vi "Read Std Dev.vi"(8 "error in (no error)":errorcluster, 11 "Std Dev in":refnum<class "Std Dev.lvclass">) -> (0 "error out":errorcluster, 1 "Channels w/ Std Dev":string[](array[string]), 2 "4 Data Points":dbl[](array[numeric]), 3 "Std Dev out":refnum<class "Std Dev.lvclass">)   [LabVIEW 2009, in "Std Dev.lvclass"]
doc: "Returns the Standard Deviation of a readable instrument.\n\nPublic Interface for \"_Read.vi\""
uses:
  Std Dev.lvclass
  Std Dev.lvclass/Std Dev.ctl
  Readable/Readable.lvclass
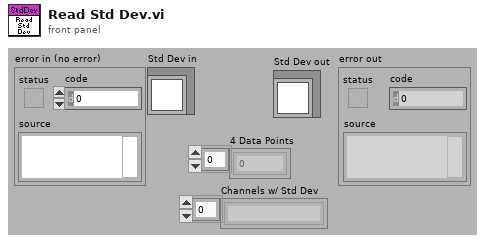
[diagram p1: front panel]
types:
  T1 = typedef "Readable.lvclass/Channel Names.ctl" = string[]
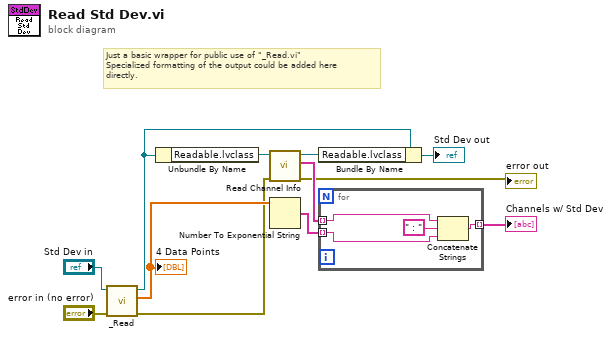
[diagram p0: block diagram]
diagram:
  # "Just a basic wrapper for public use of \"_Read.vi\"\nSpecialized formatting of the output could be added here\ndirectly."
  n1 = call-dynamic "_Read.vi"("error in (no error)"="error in (no error)", "Std Dev in"="Std Dev in") -> ("error out"=w1:errorcluster, "4 Data Points"=w11:dbl[], "Std Dev out"=w6:refnum<class "Std Dev.lvclass">)  [unwired: 7 in]
  "4 Data Points" <- w11
  n2 = Unbundle By Name(w6) -> ("Readable.lvclass"=w9:refnum<class "Readable.lvclass">)
  n3 = call "Read Channel Info.vi"("error in (no error)"=w1, "Readable.lvclass in"=w9) -> ("error out"=→"error out":errorcluster, "Channel Names"=w3:T1, "Readable.lvclass out"=w8:refnum<class "Readable.lvclass">)  [unwired: 5 in, 2 out]
  n4 = Number To Exponential String(number=w11) -> (E-format string=w5:string[])  [unwired: 3 in]
  n5 = Bundle By Name(cluster=w6, "Readable.lvclass"=w8) -> (→"Std Dev out":refnum<class "Std Dev.lvclass">)
  n6 = for {
    tunnel: w5 -> [w14] mode=indexing
    tunnel: w3 -> [w15] mode=indexing
    tunnel: [w16] -> w4 mode=indexing
    n7 = Concatenate Strings(w15, " : " ("string"), w14) -> (w16:string)
  }
  "Channels w/ Std Dev" <- w4
